vi "INSERT Multivalue.vi"(6 "Array":timestamp[](array[timestamp]), 8 "error in":errorcluster, 9 "Data":variant, 10 "Path(s)":variant, 11 "Data.PG in":refnum<class "LV-Data.PGSQL.lvclass">) -> (0 "error out":errorcluster, 1 "Wrote All to DB?":bool, 2 "Paths out":string, 3 "Data.PG out":refnum<class "LV-Data.PGSQL.lvclass">)   [LabVIEW 2019, in "LV-Data.PGSQL.lvclass"]
uses:
  LV-Data.PGSQL.lvclass
  Typedefs/Errors--enum.ctl
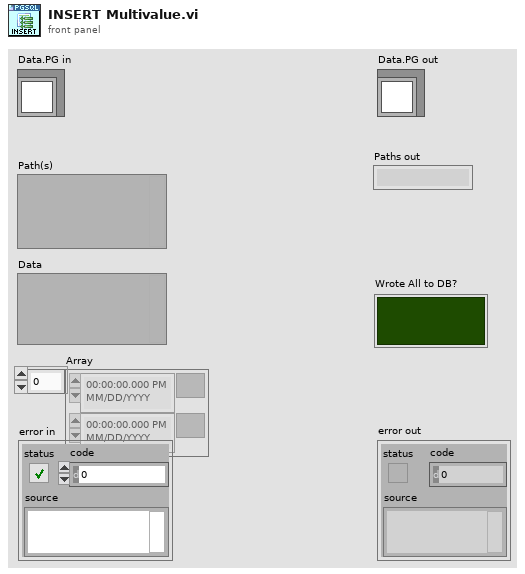
[diagram p1: front panel]
types:
  T1 = typedef "LV-Data.PGSQL.lvclass/Errors--enum.ctl" = enum16{"0: None", "5005: Path Type Not Supported", "5006: Number of Variables", "5007: Number of data points", "5008: Cannot write two data points", "5030: Start and End Times Identical", "5031: Input is not wholly", "5032: Undefined Timestamps", "5033: Bad path or paths", "5040: Invalid Instrument Name", "5050: Column can only hold string", "5051: Column can only hold bool", "5052: Column can only hold double", "5053: Column can only hold int"}
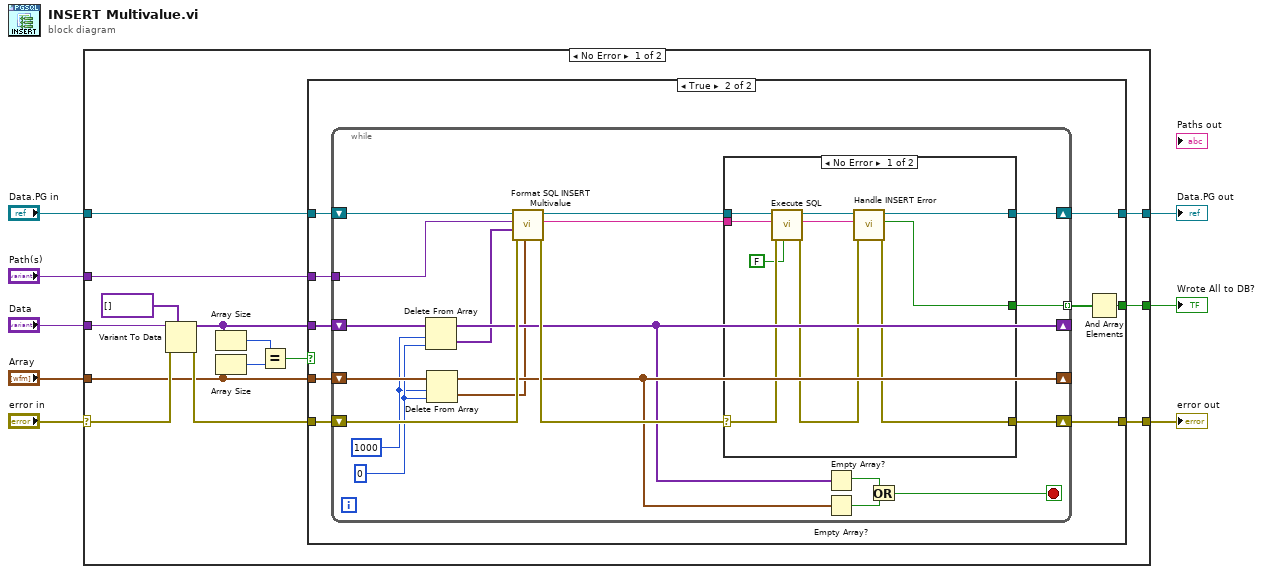
[diagram p0: block diagram]
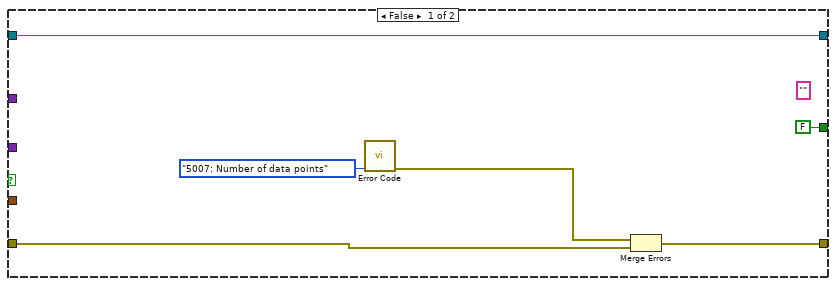
[diagram p2: hidden frame]
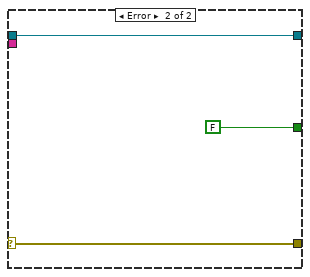
[diagram p3: hidden frame]
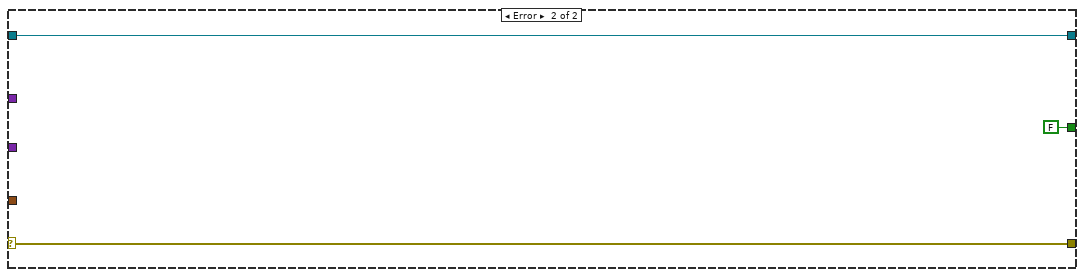
[diagram p4: hidden frame]
diagram:
  n1 = case shown="No Error" "error in" {
    selector: "error in" -> [w17 w72]
    tunnel: [w22 w72] -> w8
    tunnel: "Data.PG in" -> [w21 w71]
    tunnel: [w20 w71] -> w6
    tunnel: "Path(s)" -> [w19 _]
    tunnel: "Data" -> [w18 _]
    tunnel: [w14 FALSE] -> w2
    tunnel: "Array" -> [w12 _]
    frame No Error {
      n2 = Variant To Data(error in=w17, type=variant[] [], Variant=w18) -> (data=w13:variant[], error out=w16:errorcluster)
      n3 = Array Size(array=w13) -> (size(s)=w10:i32)
      n4 = Array Size(array=w12) -> (size(s)=w11:i32)
      n5 = Equal?(x=w10, y=w11) -> (x = y?=w9:bool)
      n6 = case shown="True" w9 {
        tunnel: [w23 w37] -> w22
        tunnel: w21 -> [w27 w36]
        tunnel: [w27 w35] -> w20
        tunnel: w19 -> [_ w34]
        tunnel: w16 -> [w24 w33]
        tunnel: [FALSE w31] -> w14
        tunnel: w13 -> [_ w30]
        tunnel: w12 -> [_ w29]
        frame False {
          (unwired) "" ("Paths out")
          n7 = call "Error Code.vi"("Error code"=Errors--enum."5007: Number of data points") -> ("error out"=w25:errorcluster)  [unwired: 10 in]
          n8 = Merge Errors(w25, w24) -> (w23:errorcluster)
        }
        frame True {
          n9 = while {
            tunnel: [w57] -> w32 mode=indexing
            tunnel: w34 -> [w40]
            shift-right: [w53] -> w37
            shift-left: w33 -> [w55]
            shift-right: [w52] -> w35
            shift-left: w36 -> [w39]
            shift-right: [w46] -> _
            shift-left: w30 -> [w51]
            shift-right: [w47] -> _
            shift-left: w29 -> [w50]
            stop <- w43 stop-if-true
            w49 = 0 ("index")
            w48 = 1000 ("length")
            n10 = Delete From Array(array=w51, length=w48, index=w49) -> (deleted portion=w41:variant[], array with subset deleted=w46:variant[])
            n11 = Delete From Array(array=w50, length=w48, index=w49) -> (deleted portion=w42:timestamp[], array with subset deleted=w47:timestamp[])
            n12 = call "Format SQL INSERT Multivalue.vi"("Times"=w42, "error in"=w55, "Data"=w41, "Path(s)"=w40, "Data.PG in"=w39) -> ("error out"=w56:errorcluster, "SQL"=w54:string, "Data.PG out"=w38:refnum<class "LV-Data.PGSQL.lvclass">)  [unwired: 3 in, 1 out]
            n13 = case shown="No Error" w56 {
              selector: w56 -> [w61 w67]
              tunnel: [w60 w67] -> w53
              tunnel: w38 -> [w64 w69]
              tunnel: [w66 w69] -> w52
              tunnel: [w65 FALSE] -> w57
              tunnel: w54 -> [w59 _]
              frame No Error {
                n14 = call "Execute SQL.vi"("Result?"=FALSE, "error in"=w61, "SQL"=w59, "LV-Data.PGSQL"=w64) -> ("error out"=w62:errorcluster, "LV-Data.PGSQL out"=w63:refnum<class "LV-Data.PGSQL.lvclass">)  [unwired: 4 in, 2 out]
                n15 = call "Handle INSERT Error.vi"("error in (no error)"=w62, "SQL"=w59, "Database.PG"=w63) -> ("error out"=w60:errorcluster, "Wrote to DB?"=w65:bool, "Database.PG out"=w66:refnum<class "LV-Data.PGSQL.lvclass">)  [unwired: 6 in]
              }
              frame Error {
              }
            }
            n16 = Empty Array?(array=w46) -> (empty?=w45:bool)
            n17 = Empty Array?(array=w47) -> (empty?=w44:bool)
            n18 = Or(x=w45, y=w44) -> (x .or. y?=w43:bool)
          }
          n19 = And Array Elements(Boolean array=w32) -> (logical AND=w31:bool)
        }
      }
    }
    frame Error {
    }
  }
  "error out" <- w8
  "Data.PG out" <- w6
  "Wrote All to DB?" <- w2
